vi "String to QAM Data.vi"(8 "error in (no error)":errorcluster, 10 "Mode":T1, 11 "Transmitted Data String":string) -> (0 "error out":errorcluster, 2 "symbol map 16 QAM":cdb[](array[numeric]), 3 "QAM Data":cluster{dbl[], dbl[]})   [LabVIEW 2011]
uses:
  Wifi Test Modes.ctl
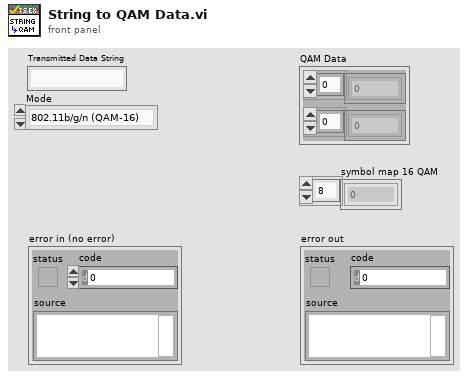
[diagram p1: front panel]
types:
  T1 = typedef "Wifi Test Modes.ctl" = enum16{"802.11b/g/n (QAM-16)", "LTE (QAM-64)", "802.11ac (QAM-256)"}
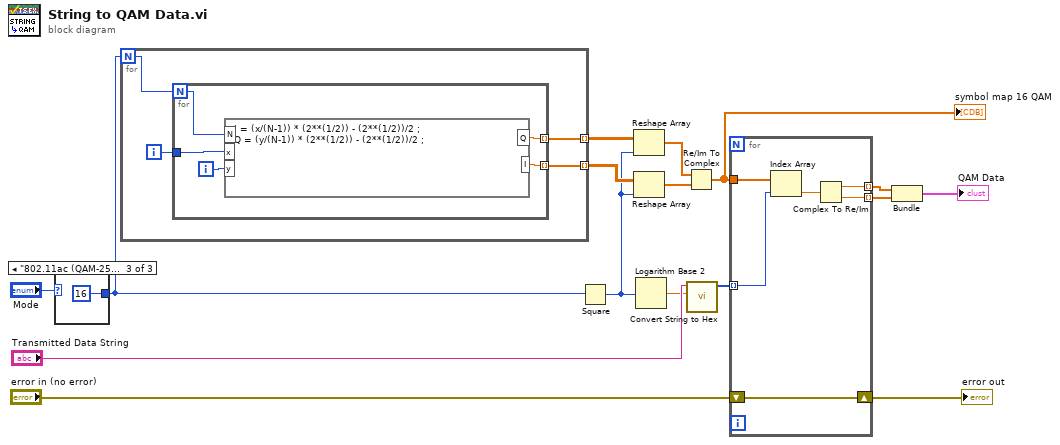
[diagram p0: block diagram]
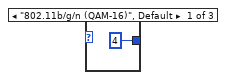
[diagram p2: hidden frame]
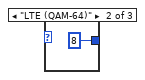
[diagram p3: hidden frame]
diagram:
  n1 = case shown="\"802.11ac (QAM-256)\"" "Mode" {
    tunnel: [4 8 16] -> w1
    frame "802.11b/g/n (QAM-16)", Default {
    }
    frame "LTE (QAM-64)" {
    }
    frame "802.11ac (QAM-256)" {
    }
  }
  n2 = for {
    N: w1 -> [w23]
    tunnel: [w21] -> w10 mode=indexing
    tunnel: [w20] -> w11 mode=indexing
    i -> [w22]
    n3 = for {
      N: w23 -> [w28]
      tunnel: w22 -> [w27]
      tunnel: [w25] -> w21 mode=indexing
      tunnel: [w24] -> w20 mode=indexing
      i -> [w26]
      n4 = formula code="I = (x/(N-1)) * (2**(1/2)) - (2**(1/2))/2 ;\nQ = (y/(N-1)) * (2**(1/2)) - (2**(1/2))/2 ;"("x"=w27, "y"=w26, "N"=w28) -> ("Q"=w25:dbl, "I"=w24:dbl)
    }
  }
  n5 = Square(x=w1) -> (x^2=w3:i32)
  n6 = Reshape Array(w10, w3) -> (w8:dbl[])
  n7 = Reshape Array(w11, w3) -> (w9:dbl[])
  n8 = Logarithm Base 2(1:w3) -> (0:w4:dbl)
  n9 = Re/Im To Complex(1:w9, 2:w8) -> (0:w2:cdb[])
  "symbol map 16 QAM" <- w2
  n10 = call "Convert String to Hex.vi"("bits per element"=w4, "Input String"="Transmitted Data String") -> ("Hex Values"=w13:u8[])  [unwired: 8 in]
  n11 = for {
    tunnel: w2 -> [w33]
    tunnel: [w30] -> w6 mode=indexing
    tunnel: [w29] -> w7 mode=indexing
    tunnel: w13 -> [w32] mode=indexing
    shift-right: [w31] -> w15
    shift-left: "error in (no error)" -> [w31]
    n12 = Index Array(array=w33, index=w32) -> (element=w34:cdb)
    n13 = Complex To Re/Im(x + iy=w34) -> (x=w30:dbl, y=w29:dbl)
  }
  "error out" <- w15
  n14 = Bundle(w6, w7) -> (→"QAM Data":cluster{dbl[], dbl[]})  [unwired: 1 in]
